vi "read one data transmit.vi"(0 "Serial Port":refnum<visa-resource-name>, 2 "2nd channel":bool) -> (1 "got data":bool, 3 "Temperature":sgl format="%.2f", 4 "Channel 2":sgl format="%.2f", 5 "Sample ID":u32, 6 "Channel 1 units":string, 7 "Channel 1 label":string, 8 "Channel 1":sgl format="%.2f", 9 "Channel 2 units":string, 10 "Channel 2 label":string)   [LabVIEW 2010]
panel:
  out "chars":dbl format="%.2f"
  out "chars":dbl format="%.2f"
  out "reply":string
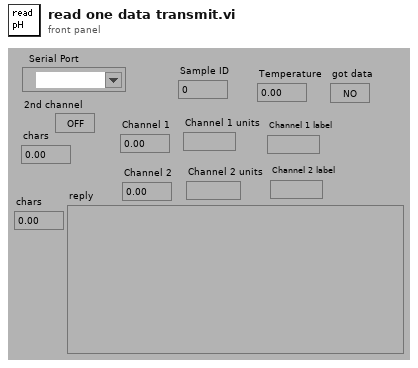
[diagram p1: front panel]
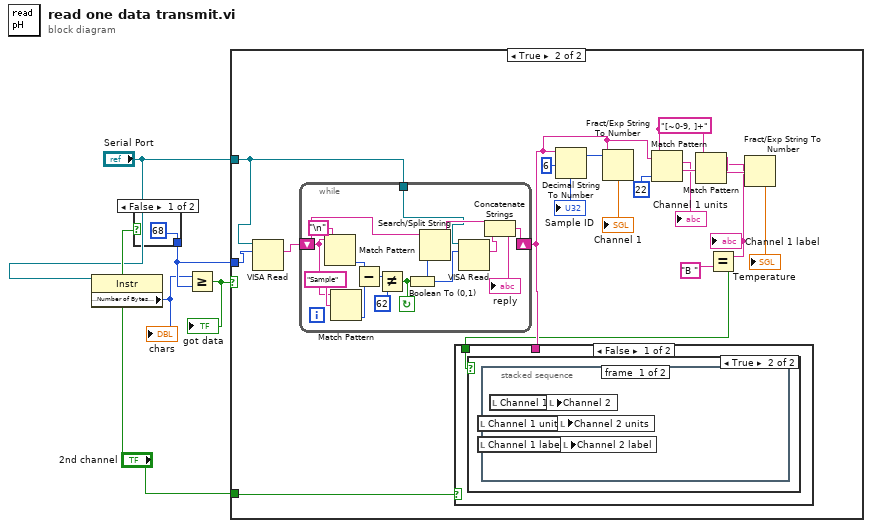
[diagram p0: block diagram]
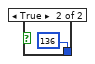
[diagram p2: hidden frame]
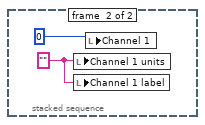
[diagram p5: hidden frame]
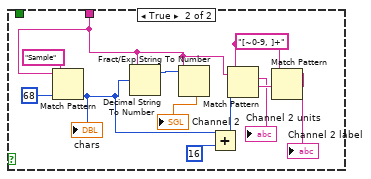
[diagram p6: hidden frame]
diagram:
  n1 = property class="Instr"(reference="Serial Port") -> ("Serial Settings:Number of Bytes at Serial Port"=w1:u32)  [unwired: 1 in, 2 out]
  "chars" <- w1
  n2 = case shown="False" "2nd channel" {
    tunnel: [68 136] -> w3
    frame False {
    }
    frame True {
    }
  }
  n3 = Greater Or Equal?(x=w1, y=w3) -> (x >= y?=w5:bool)
  "got data" <- w5
  n4 = case shown="True" w5 {
    tunnel: "Serial Port" -> [_ w9]
    tunnel: "2nd channel" -> [_ w14]
    tunnel: w3 -> [_ w10]
    frame False {
    }
    frame True {
      w18 = "[~0-9, ]+"
      n5 = VISA Read(VISA resource name=w9, byte count=w10) -> (read buffer=w8:string)  [unwired: 1 in, 3 out]
      n6 = while {
        shift-left: w8 -> [w32]
        shift-right: [w36] -> w24
        tunnel: w9 -> [w28]
        stop <- w29 continue-if-true
        n7 = Match Pattern(string=w32, regular expression="\n") -> (offset past match=w30:i32)  [unwired: 1 in, 3 out]
        n8 = Match Pattern(string=w32, regular expression="Sample") -> (offset past match=w34:i32)  [unwired: 1 in, 3 out]
        n9 = Subtract(x=w30, y=w34) -> (x-y=w31:i32)
        n10 = Not Equal?(x=w31, y=62) -> (x != y?=w29:bool)
        n11 = Boolean To (0,1)(Boolean=w29) -> (0, 1=w27:i16)
        n12 = Search/Split String(string=w32, offset (0)=w27) -> (match + rest of string=w33:string)  [unwired: 1 in, 2 out]
        n13 = VISA Read(VISA resource name=w28, byte count=w27) -> (read buffer=w26:string)  [unwired: 1 in, 3 out]
        n14 = Concatenate Strings(w33, w26) -> (w36:string)
        "reply" <- w36
      }
      n15 = Decimal String To Number(string=w24, offset=6) -> (offset past number=w16:i32, number=→"Sample ID":i32)  [unwired: 1 in]
      n16 = Fract/Exp String To Number(string=w24, offset=w16) -> (number=→"Channel 1":dbl)  [unwired: 2 in, 1 out]
      n17 = Match Pattern(string=w24, regular expression=w18, offset (0)=22) -> (match substring=→"Channel 1 units":string, after substring=w21:string)  [unwired: 2 out]
      n18 = Match Pattern(string=w21, regular expression=w18) -> (match substring=w13:string, after substring=w23:string)  [unwired: 1 in, 2 out]
      "Channel 1 label" <- w13
      n19 = Equal?(x=w13, y="B ") -> (x = y?=w11:bool)
      n20 = case shown="False" w14 {
        tunnel: w24 -> [_ w48]
        tunnel: w11 -> [w39 _]
        frame False {
          n21 = case shown="True" w39 {
            frame False {
            }
            frame True {
              n22 = stacked-sequence {
                frame #0 {
                  n23 = local read "Channel 1 units"() -> (w41:string)
                  n24 = local read "Channel 1 label"() -> (w40:string)
                  n25 = local read "Channel 1"() -> (w42:sgl)
                  n26 = local write "Channel 2"(w42) -> ()
                  n27 = local write "Channel 2 units"(w41) -> ()
                  n28 = local write "Channel 2 label"(w40) -> ()
                }
                frame #1 {
                  w43 = ""
                  n29 = local write "Channel 1 units"(w43) -> ()
                  n30 = local write "Channel 1 label"(w43) -> ()
                  n31 = local write "Channel 1"(0) -> ()
                }
              }
            }
          }
        }
        frame True {
          w55 = "[~0-9, ]+"
          n32 = Match Pattern(string=w48, regular expression="Sample", offset (0)=68) -> (offset past match=w45:i32)  [unwired: 3 out]
          "chars" <- w45
          n33 = Decimal String To Number(string=w48, offset=w45) -> (offset past number=w54:i32)  [unwired: 1 in, 1 out]
          n34 = Fract/Exp String To Number(string=w48, offset=w54) -> (number=→"Channel 2":dbl)  [unwired: 2 in, 1 out]
          n35 = Add(x=w45, y=16) -> (x+y=w47:i32)
          n36 = Match Pattern(string=w48, regular expression=w55, offset (0)=w47) -> (match substring=→"Channel 2 units":string, after substring=w56:string)  [unwired: 2 out]
          n37 = Match Pattern(string=w56, regular expression=w55) -> (match substring=→"Channel 2 label":string)  [unwired: 1 in, 3 out]
        }
      }
      n38 = Fract/Exp String To Number(string=w23) -> (number=→"Temperature":dbl)  [unwired: 3 in, 1 out]
    }
  }
